vi "Timeout Thinking.vi"(8 "error in (no error)":errorcluster, 11 "Philosopher in":refnum<class "Philosopher.lvclass">) -> (0 "error out":errorcluster, 3 "Philosopher out":refnum<class "Philosopher.lvclass">)   [LabVIEW 2023, in "Philosopher.lvlib" / "Philosopher.lvclass"]
uses:
  Philosopher.lvclass
  C:/Program Files (x86)/National Instruments/LabVIEW 2023/vi.lib/ActorFramework/Actor/Actor.lvclass
  <vilib>/ActorFramework/Actor/Actor.lvclass/Actor.ctl
  Philosopher.lvclass/Philosopher.ctl
  Table/Table Messages/Hungry Msg/Hungry Msg.lvclass/Hungry Msg.ctl
  <vilib>/ActorFramework/Message Enqueuer/Message Enqueuer.lvclass/Message Enqueuer.ctl
  <vilib>/ActorFramework/Message Enqueuer/Enqueue.vi
  Table/Table Messages/Hungry Msg/Hungry Msg.lvclass
  C:/Program Files (x86)/National Instruments/LabVIEW 2023/vi.lib/ActorFramework/Message/Message.lvclass
  <vilib>/Utility/LVClass/Get LV Class Name.vi
  <resource>/AFDebug/Generate Trace for Message.vi
  <vilib>/ActorFramework/Message Priority Queue/Priority Enqueue.vi
  <vilib>/ActorFramework/Actor/Actor.lvclass
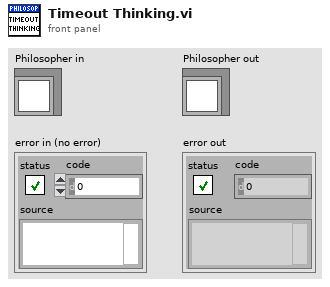
[diagram p1: front panel]
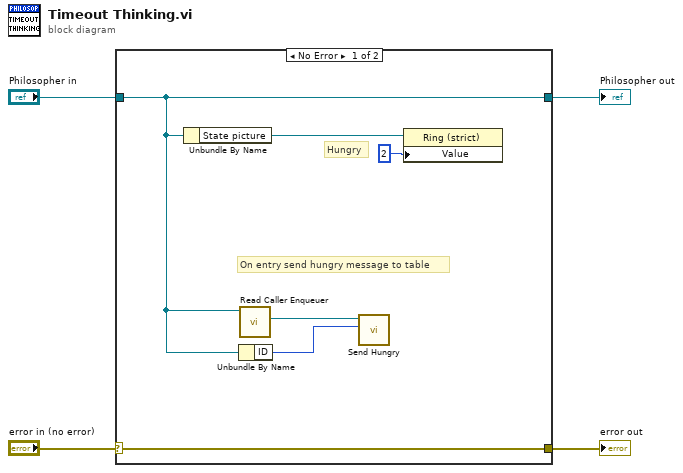
[diagram p0: block diagram]
diagram:
  n1 = case shown="No Error" "error in (no error)" {
    selector: "error in (no error)" -> [w10 w12]
    tunnel: [w10 w12] -> w3
    tunnel: [w7 w11] -> w1
    tunnel: "Philosopher in" -> [w7 w11]
    frame No Error {
      # "Hungry"
      # "On entry send hungry message to table"
      n2 = Unbundle By Name(w7) -> ("State picture"=w9:refnum<vi>)
      n3 = Unbundle By Name(w7) -> ("ID"=w6:i32)
      n4 = call <vilib>:"Read Caller Enqueuer.vi"("Actor"=w7) -> ("Caller Enqueuer"=w8:refnum<class "Message Enqueuer.lvclass">)  [unwired: 10 in]
      n5 = call "Send Hungry.vi"("Philosopher ID"=w6, "Message Enqueuer"=w8) -> ()  [unwired: 8 in, 2 out]
      n6 = property class="Ring (strict)"(reference=w9, "Value"=2) -> ()  [unwired: 1 in, 2 out]
    }
    frame Error {
    }
  }
  "error out" <- w3
  "Philosopher out" <- w1
